vi "Arduino Response List_MI.vi"(11 "MachineInterfaceRecipeOpcodes":T1) -> (0 "Number of Racks":i32, 1 "Rack2 Response":T3, 2 "Rack1 Response":T3, 3 "Ping Response, Button Press, Incorrect Opcode":T2)   [LabVIEW 2019, in "Machine Interface.lvclass"]
uses:
  Machine Interface.lvclass
  Controls/Machine Interface Config File Structure_MI.ctl
  Controls/Response from Hardware_MI.ctl
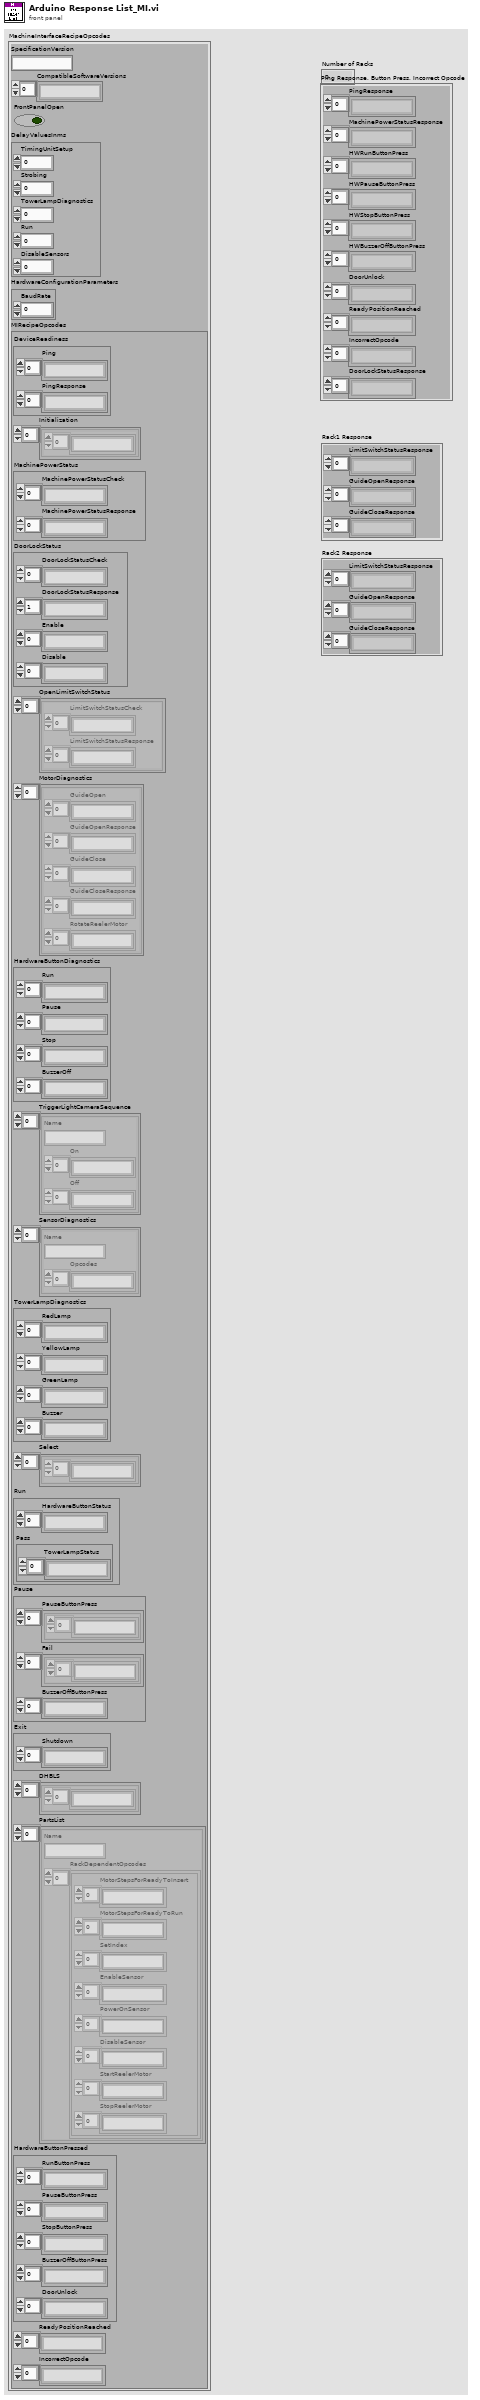
[diagram p1: front panel]
types:
  T1 = typedef "Machine Interface.lvclass/Machine Interface Config File Structure_MI.ctl" = cluster{"SpecificationVersion":string, "CompatibleSoftwareVersions":string[], "FrontPanelOpen":bool, "DelayValuesInms":cluster{"TimingUnitSetup":i32, "Strobing":i32, "TowerLampDiagnostics":i32, "Run":i32, "DisableSensors":i32}, "HardwareConfigurationParameters":cluster{"BaudRate":dbl}, "MIRecipeOpcodes":cluster{"DeviceReadiness":cluster{"Ping":string[], "PingResponse":string[]}, "Initialization":cluster{string[]}[], "MachinePowerStatus":cluster{"MachinePowerStatusCheck":string[], "MachinePowerStatusResponse":string[]}, "DoorLockStatus":cluster{"DoorLockStatusCheck":string[], "DoorLockStatusResponse":string[], "Enable":string[], "Disable":string[]}, "OpenLimitSwitchStatus":cluster{"LimitSwitchStatusCheck":string[], "LimitSwitchStatusResponse":string[]}[], "MotorDiagnostics":cluster{"GuideOpen":string[], "GuideOpenResponse":string[], "GuideClose":string[], "GuideCloseResponse":string[], "RotateReelerMotor":string[]}[], "HardwareButtonDiagnostics":cluster{"Run":string[], "Pause":string[], "Stop":string[], "BuzzerOff":string[]}, "TriggerLightCameraSequence":cluster{"Name":string, "On":string[], "Off":string[]}[], "SensorDiagnostics":cluster{"Name":string, "Opcodes":string[]}[], "TowerLampDiagnostics":cluster{"RedLamp":string[], "YellowLamp":string[], "GreenLamp":string[], "Buzzer":string[]}, "Select":cluster{string[]}[], "Run":cluster{"HardwareButtonStatus":string[], "Pass":cluster{"TowerLampStatus":string[]}}, "Pause":cluster{"PauseButtonPress":cluster{string[]}[], "Fail":cluster{string[]}[], "BuzzerOffButtonPress":string[]}, "Exit":cluster{"Shutdown":string[]}, "DHBLS":cluster{string[]}[], "PartsList":cluster{"Name":string, "RackDependentOpcodes":cluster{"MotorStepsForReadyToInsert":string[], "MotorStepsForReadyToRun":string[], "SetIndex":string[], "EnableSensor":string[], "PowerOnSensor":string[], "DisableSensor":string[], "StartReelerMotor":string[], "StopReelerMotor":string[]}[]}[], "HardwareButtonPressed":cluster{"RunButtonPress":string[], "PauseButtonPress":string[], "StopButtonPress":string[], "BuzzerOffButtonPress":string[], "DoorUnlock":string[]}, "ReadyPositionReached":string[], "IncorrectOpcode":string[]}}
  T2 = typedef "Machine Interface.lvclass/Response from Hardware_MI.ctl" = cluster{"PingResponse":string[], "MachinePowerStatusResponse":string[], "HWRunButtonPress":string[], "HWPauseButtonPress":string[], "HWStopButtonPress":string[], "HWBuzzerOffButtonPress":string[], "DoorUnlock":string[], "ReadyPositionReached":string[], "IncorrectOpcode":string[], "DoorLockStatusResponse":string[]}
  T3 = cluster{"LimitSwitchStatusResponse":string[], "GuideOpenResponse":string[], "GuideCloseResponse":string[]}
  T4 = cluster{"LimitSwitchStatusCheck":string[], "LimitSwitchStatusResponse":string[]}[]
  T5 = cluster{"GuideOpen":string[], "GuideOpenResponse":string[], "GuideClose":string[], "GuideCloseResponse":string[], "RotateReelerMotor":string[]}[]
  T6 = cluster{"PingResponse":string[], "MachinePowerStatusResponse":string[], "RunButtonPress":string[], "PauseButtonPress":string[], "StopButtonPress":string[], "BuzzerOffButtonPress":string[], "DoorUnlock":string[], "ReadyPositionReached":string[], "IncorrectOpcode":string[], "DoorLockStatusResponse":string[]}
  T7 = cluster{"LimitSwitchStatusCheck":string[], "LimitSwitchStatusResponse":string[]}
  T8 = cluster{"GuideOpen":string[], "GuideOpenResponse":string[], "GuideClose":string[], "GuideCloseResponse":string[], "RotateReelerMotor":string[]}
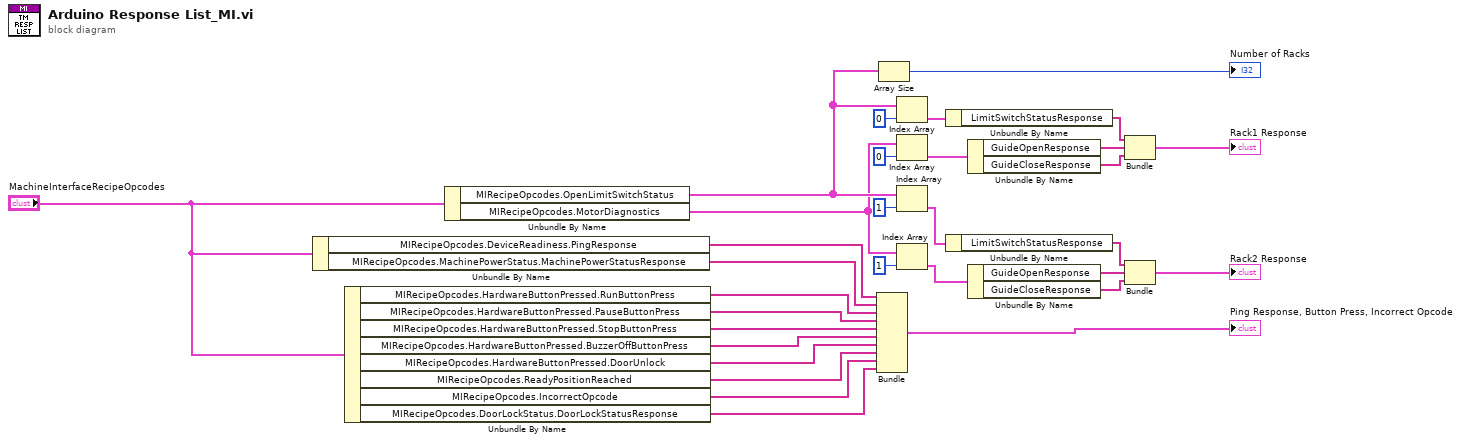
[diagram p0: block diagram]
diagram:
  n1 = Unbundle By Name("MachineInterfaceRecipeOpcodes") -> ("MIRecipeOpcodes.DeviceReadiness.PingResponse"=w31:string[], "MIRecipeOpcodes.MachinePowerStatus.MachinePowerStatusResponse"=w5:string[])
  n2 = Unbundle By Name("MachineInterfaceRecipeOpcodes") -> ("MIRecipeOpcodes.HardwareButtonPressed.RunButtonPress"=w7:string[], "MIRecipeOpcodes.HardwareButtonPressed.PauseButtonPress"=w8:string[], "MIRecipeOpcodes.HardwareButtonPressed.StopButtonPress"=w9:string[], "MIRecipeOpcodes.HardwareButtonPressed.BuzzerOffButtonPress"=w10:string[], "MIRecipeOpcodes.HardwareButtonPressed.DoorUnlock"=w2:string[], "MIRecipeOpcodes.ReadyPositionReached"=w11:string[], "MIRecipeOpcodes.IncorrectOpcode"=w30:string[], "MIRecipeOpcodes.DoorLockStatus.DoorLockStatusResponse"=w1:string[])
  n3 = Unbundle By Name("MachineInterfaceRecipeOpcodes") -> ("MIRecipeOpcodes.OpenLimitSwitchStatus"=w29:T4, "MIRecipeOpcodes.MotorDiagnostics"=w28:T5)
  n4 = Bundle("PingResponse"=w31, "MachinePowerStatusResponse"=w5, "RunButtonPress"=w7, "PauseButtonPress"=w8, "StopButtonPress"=w9, "BuzzerOffButtonPress"=w10, "DoorUnlock"=w2, "ReadyPositionReached"=w11, "IncorrectOpcode"=w30, "DoorLockStatusResponse"=w1) -> (→"Ping Response, Button Press, Incorrect Opcode":T6)  [unwired: 1 in]
  n5 = Array Size(array=w29) -> (size(s)=→"Number of Racks":i32)
  n6 = Index Array(array=w29, index=0) -> (element=w13:T7)
  n7 = Index Array(array=w28, index=0) -> (element=w15:T8)
  n8 = Index Array(array=w29, index=1) -> (element=w21:T7)
  n9 = Index Array(array=w28, index=1) -> (element=w23:T8)
  n10 = Unbundle By Name(w13) -> ("LimitSwitchStatusResponse"=w16:string[])
  n11 = Unbundle By Name(w21) -> ("LimitSwitchStatusResponse"=w24:string[])
  n12 = Unbundle By Name(w15) -> ("GuideOpenResponse"=w18:string[], "GuideCloseResponse"=w17:string[])
  n13 = Unbundle By Name(w23) -> ("GuideOpenResponse"=w26:string[], "GuideCloseResponse"=w25:string[])
  n14 = Bundle("LimitSwitchStatusResponse"=w16, "GuideOpenResponse"=w18, "GuideCloseResponse"=w17) -> (→"Rack1 Response":T3)  [unwired: 1 in]
  n15 = Bundle("LimitSwitchStatusResponse"=w24, "GuideOpenResponse"=w26, "GuideCloseResponse"=w25) -> (→"Rack2 Response":T3)  [unwired: 1 in]
